vi "FindRecentItem.vi"(11 "recent_item":path) -> (2 "found":bool, 3 "MetaDataObj out":refnum<class "MetaDataObj.lvclass">)   [LabVIEW 2016]
uses:
  <resource>/dialog/NewProjectWizard/MetaDataObj/MetaDataObj.lvclass
  <resource>/dialog/NewProjectWizard/MetaDataObj/Accessors/Read LocationPath.vi
  <resource>/dialog/NewProjectWizard/Loading Project Info/NI_NPW_Loading Project Info.lvlib
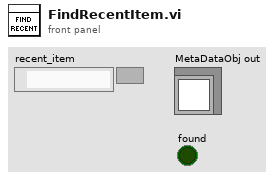
[diagram p1: front panel]
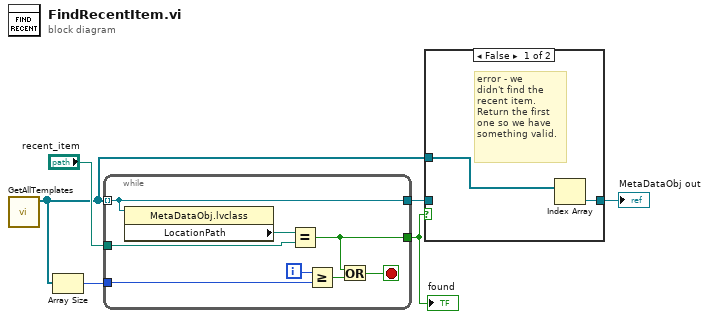
[diagram p0: block diagram]
diagram:
  n1 = call <resource>:"GetAllTemplates.vi"() -> ("Templates Out"=w1:refnum<class "MetaDataObj.lvclass">[])  [unwired: 11 in]
  n2 = Array Size(array=w1) -> (size(s)=w5:i32)
  n3 = while {
    tunnel: w1 -> [w14] mode=indexing
    tunnel: "recent_item" -> [w12]
    tunnel: [w14] -> w4
    tunnel: w5 -> [w10]
    tunnel: [w7] -> w2
    i -> [w11]
    stop <- w8 stop-if-true
    n4 = property class="MetaDataObj.lvclass"(reference=w14) -> ("LocationPath"=w13:path)  [unwired: 1 in, 2 out]
    n5 = Equal?(x=w13, y=w12) -> (x = y?=w7:bool)
    n6 = Greater Or Equal?(x=w11, y=w10) -> (x >= y?=w9:bool)
    n7 = Or(x=w7, y=w9) -> (x .or. y?=w8:bool)
  }
  "found" <- w2
  n8 = case shown="False" w2 {
    tunnel: w4 -> [_ w17]
    tunnel: [w15 w17] -> w3
    tunnel: w1 -> [w16 _]
    frame False {
      # "error - we\ndidn't find the\nrecent item.\nReturn the first\none so we have\nsomething valid."
      n9 = Index Array(array=w16) -> (element=w15:refnum<class "MetaDataObj.lvclass">)  [unwired: 1 in]
    }
    frame True {
    }
  }
  "MetaDataObj out" <- w3
